vi "timesensorvariable.vi"(9 "Elapsed time in current state":dbl format="%.2f", 10 "S P & V definitions":T3[](array[typedef]) {"value" format="%#_6p"; "variable"."Data average interval" min=0.0 format="%^#_3g"}, 11 "condition":T1 {"Data average interval" min=0.0 format="%^#_3g"; "sensors and variables" items=["Elapsed time in current state"]}) -> (3 "exit":bool)   [LabVIEW 2012]
uses:
  variable setpoint.ctl
  data ave interval.ctl
  type specifier for control code.ctl
  condition.ctl
  greater or less.ctl
  DAQ configuration/Sensor buffer command.ctl
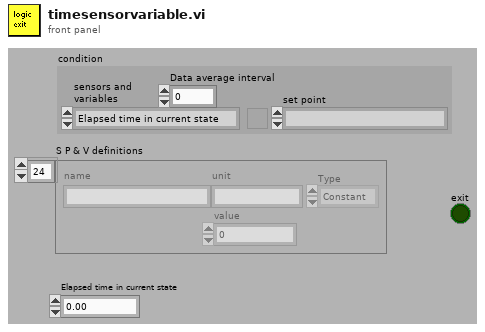
[diagram p1: front panel]
types:
  T1 = typedef "condition.ctl" = cluster{"> or <":T2, "set point":i32, "sensors and variables":i32, "Data average interval":dbl}
  T2 = typedef "greater or less.ctl" = bool
  T3 = typedef "variable setpoint.ctl" = cluster{"name":string, "unit":string, "value":dbl, "Type":enum16{"Constant", "Variable"}, "variable":cluster{"selected sensors":i32[], "selected set points":i32[], "VI":path, "Data average interval":T4, "code ref":T5}}
  T4 = typedef "data ave interval.ctl" = dbl
  T5 = typedef "type specifier for control code.ctl" = refnum<vi>
  T6 = typedef "Sensor buffer command.ctl" = enum16{"read average", "read recent", "read all", "write", "configure", "clear"}
  T7 = typedef "Sensor data.ctl" = cluster{" Sensor array":T8[], "Time":dbl}
  T8 = typedef "sensor cluster.ctl" = cluster{"voltage":sgl, "scaled":sgl, "units":string, "Out of Range":bool}
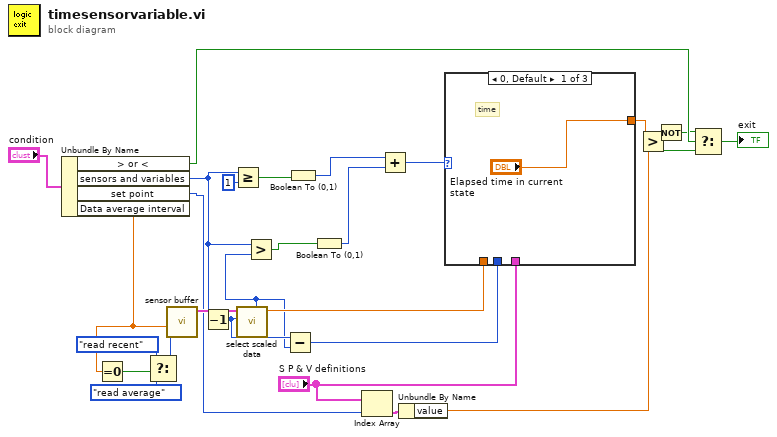
[diagram p0: block diagram]
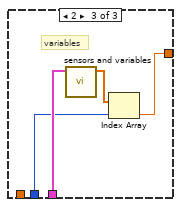
[diagram p3: hidden frame]
diagram:
  n1 = Unbundle By Name("condition") -> ("> or <"=w12:T2, "sensors and variables"=w18:i32, "set point"=w15:i32, "Data average interval"=w20:dbl)
  n2 = Equal To 0?(x=w20) -> (x = 0?=w26:bool)
  n3 = Select(t=Sensor_buffer_command."read recent" ("command"), s=w26, f=Sensor_buffer_command."read average" ("command")) -> (s? t:f=w25:T6)
  n4 = call "sensor buffer.vi"("command"=w25, "smooth interval (s)"=w20) -> ("Sensor Data smoothed"=w24:T7)  [unwired: 3 in, 2 out]
  n5 = Decrement(x=w18) -> (x-1=w5:i32)
  n6 = Greater Or Equal?(x=w18, y=1) -> (x >= y?=w27:bool)
  n7 = call "select scaled data.vi"("Sensor index"=w5, "Sensor Data"=w24) -> ("scaled"=w19:sgl, "number of sensors"=w4:i32)  [unwired: 4 in, 4 out]
  n8 = Greater?(x=w18, y=w4) -> (0:w1:bool)
  n9 = Subtract(x=w5, y=w4) -> (x-y=w3:i32)
  n10 = Boolean To (0,1)(Boolean=w27) -> (0, 1=w9:i16)
  n11 = Boolean To (0,1)(Boolean=w1) -> (0, 1=w8:i16)
  n12 = Index Array(array="S P & V definitions", index=w15) -> (element=w17:T3)
  n13 = Add(x=w9, y=w8) -> (x+y=w2:i16)
  n14 = Unbundle By Name(w17) -> ("value"=w14:dbl)
  n15 = case shown="0, Default" w2 {
    tunnel: w19 -> [_ w29 _]
    tunnel: ["Elapsed time in current state" w29 w32] -> w13
    tunnel: "S P & V definitions" -> [_ _ w31]
    tunnel: w3 -> [_ _ w30]
    frame 0, Default {
      # "time"
    }
    frame 1 {
      # "sensors"
    }
    frame 2 {
      # "variables"
      n16 = call "sensors and variables.vi"("S P & V definitions"=w31) -> ("Variable values"=w33:dbl[])  [unwired: 7 in, 3 out]
      n17 = Index Array(array=w33, index=w30) -> (element=w32:dbl)
    }
  }
  n18 = Greater?(x=w13, y=w14) -> (0:w7:bool)
  n19 = Not(x=w7) -> (.not. x?=w6:bool)
  n20 = Select(t=w6, s=w12, f=w7) -> (s? t:f=→"exit":bool)
